vi "Custom Freq Multiplier.vi"(7 "Number of pulses":u32=5) -> (0 "DO State":bool, 1 "Toggle Iterations":u32, 2 "Time elapsed (ticks)":u32, 3 "FIFO Read Timed Out?":bool)   [LabVIEW 2014]
uses:
  Custom Pulse 2.ctl
  <vilib>/rvi/Emulation/niFpgaEmulationIsFPGAContextNoSignature.vi
  <vilib>/rvi/Emulation/niFpgaSctlEmulationGetInTimedLoop.vi
  <vilib>/rvi/errors/niFpgaSetErrorForExecOnDevCompSimple.vi
  <vilib>/rvi/eio/common/nirviEmuReportErrorAndStop.vi
  <vilib>/rvi/DataTransferAndStorage/Container/Common/niFpgaContainerGetUniqueNameForEmu.vi
  <vilib>/rvi/FIFO/Fifo_Resource/nirvififoEmulationSetSize.vi
  <vilib>/rvi/FIFO/Fifo_Resource/nirviFifoEmulationQueueMgr.vi
  <instcachedir>/0/nirviFifoEmulationQueueMgr_E5CAEC123FF24DC58D834DCA3CDAA9B5.lvgen/nirviFifoEmulationQueueMgr_E5CAEC123FF24DC58D834DCA3CDAA9B5_001.vi
  <vilib>/rvi/FIFO/Fifo_Resource/nirvififoEmulationCreateLock.vi
  <vilib>/rvi/Emulation/niFpgaProcessEmulError.vi
  <vilib>/rvi/FIFO/Fifo_Resource/nirvififoEmulationObtainLock.vi
  <vilib>/rvi/FIFO/Fifo_Resource/nirvififoEmulationReleaseLock.vi
  <vilib>/rvi/occurrence/nirviWaitOnOccurrenceBase.vi
  <vilib>/rvi/errors/nirviReportUnexpectedCaseInternalError.vi
  <vilib>/rvi/errors/nirviReportUnexpectedCaseInternalError (U32).vi
  <vilib>/rvi/DataTransferAndStorage/Container/XNode/niFpgaContainer.xnode
  <vilib>/rvi/FIFO/Fifo_Resource/nirvififoEmulationRead.vi
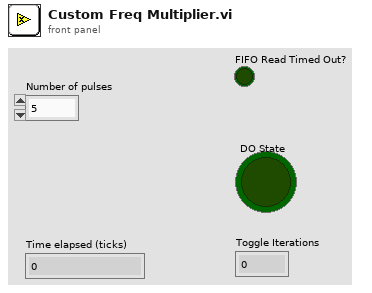
[diagram p1: front panel]
types:
  T1 = typedef "Custom Pulse 2.ctl" = enum16{"Idle", "Processing"}
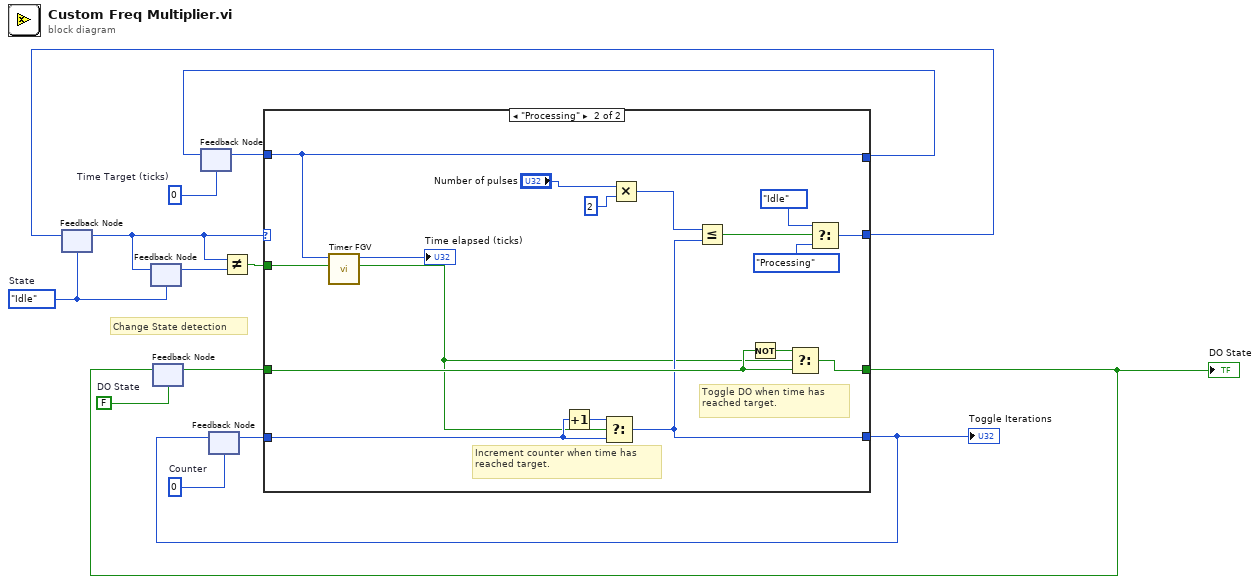
[diagram p0: block diagram]
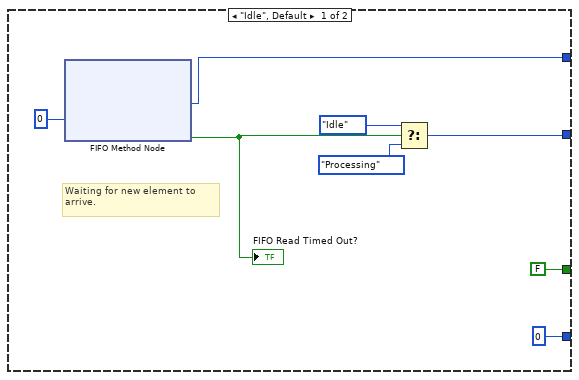
[diagram p2: hidden frame]
diagram:
  w4 = Custom_Pulse_2."Idle"  # State
  w6 = FALSE  # DO State
  w7 = u32 0  # Counter
  w8 = u32 0  # Time Target (ticks)
  # "Change State detection"
  n1 = feedback #1(w4) -> (w3:T1)
  n2 = feedback #2(w4) -> (w2:T1)
  n3 = feedback-in #2(w3) -> ()
  n4 = feedback #3(w6) -> (w11:bool)
  n5 = feedback #4(w8) -> (w14:u32)
  n6 = feedback #5(w7) -> (w13:u32)
  n7 = Not Equal?(x=w3, y=w2) -> (x != y?=w1:bool)
  n8 = case shown="\"Processing\"" w3 {
    tunnel: [w17 w27] -> w9
    tunnel: [w20 w33] -> w5
    tunnel: w14 -> [_ w27]
    tunnel: w13 -> [_ w30]
    tunnel: [u32 0 w28] -> w12
    tunnel: w11 -> [_ w37]
    tunnel: [FALSE ("DO State") w36] -> w10
    tunnel: w1 -> [_ w23]
    frame "Idle", Default {
      # "Waiting for new element to\narrive."
      n9 = xnode ("FIFO Method Node")("Timeout"=0) -> ("Element"=w17:u32, "Timed Out?"=w18:bool)  [unwired: 1 in, 1 out]
      "FIFO Read Timed Out?" <- w18
      n10 = Select(t=Custom_Pulse_2."Idle", s=w18, f=Custom_Pulse_2."Processing") -> (s? t:f=w20:T1)
    }
    frame "Processing" {
      # "Increment counter when time has\nreached target."
      # "Toggle DO when time has\nreached target."
      n11 = call "Timer FGV.vi"("Reset"=w23, "Time Target (ticks)"=w27) -> ("Time Reached?"=w26:bool, "Time elapsed (ticks)"=→"Time elapsed (ticks)":u32)  [unwired: 8 in]
      n12 = Increment(x=w30) -> (x+1=w39:u32)
      n13 = Select(t=w39, s=w26, f=w30) -> (s? t:f=w28:u32)
      n14 = Multiply(x="Number of pulses", y=u32 2) -> (x*y=w29:u32)
      n15 = Less Or Equal?(x=w29, y=w28) -> (x <= y?=w32:bool)
      n16 = Not(x=w37) -> (.not. x?=w38:bool)
      n17 = Select(t=w38, s=w26, f=w37) -> (s? t:f=w36:bool)
      n18 = Select(t=Custom_Pulse_2."Idle", s=w32, f=Custom_Pulse_2."Processing") -> (s? t:f=w33:T1)
    }
  }
  "Toggle Iterations" <- w12
  "DO State" <- w10
  n19 = feedback-in #1(w5) -> ()
  n20 = feedback-in #3(w10) -> ()
  n21 = feedback-in #4(w9) -> ()
  n22 = feedback-in #5(w12) -> ()
